vi "configMQTT.vi"(8 "error in (no error)":errorcluster, 10 "conf(empty for default)":string, 11 "Module ID":i32=-1) -> (0 "error out":errorcluster)   [LabVIEW 2017, in "ISA010_module.lvlib"]
uses:
  ISA010_module.lvlib
  libraries/MQTT.lvlibp
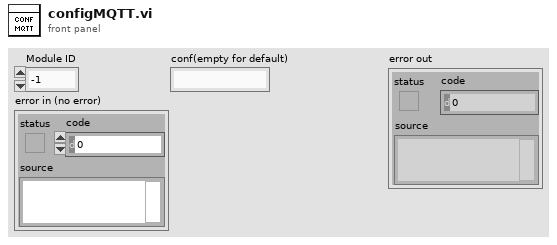
[diagram p1: front panel]
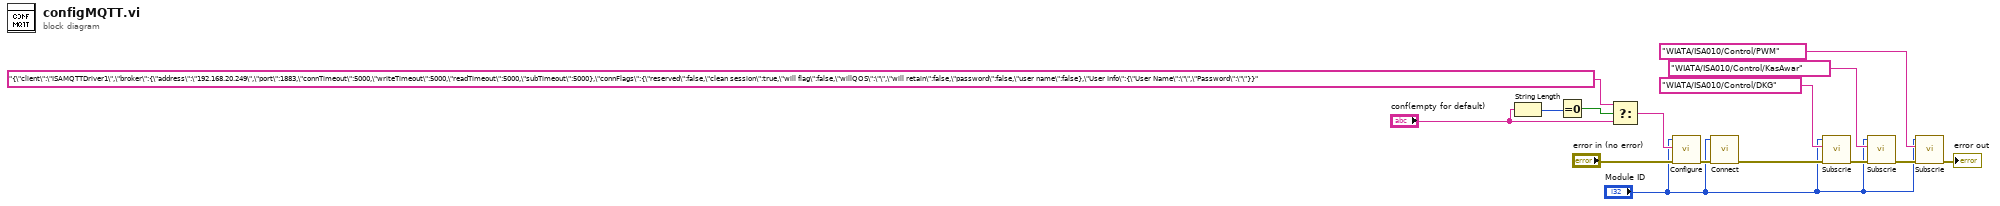
[diagram p0: block diagram]
diagram:
  n1 = String Length(string="conf(empty for default)") -> (length=w13:i32)
  n2 = Equal To 0?(x=w13) -> (x = 0?=w12:bool)
  n3 = Select(t="{\"client\":\"ISAMQTTDriver1\",\"broker\":{\"address\":\"192.168.20.249\",\"port\":1883,\"connTimeout\":5000,\"writeTimeout\":5000,\"readTimeout\":5000,\"subTimeout\":5000},\"connFlags\":{\"reserved\":false,\"clean session\":true,\"will flag\":false,\"willQOS\":\"\",\"will retain\":false,\"password\":false,\"user name\":false},\"User Info\":{\"User Name\":\"\",\"Password\":\"\"}}" ("JSON config"), s=w12, f="conf(empty for default)") -> (s? t:f=w9:string)
  n4 = call "Configure.vi"("error in (no error)"="error in (no error)", "JSON config"=w9, "Module ID"="Module ID") -> ("error out"=w15:errorcluster)  [unwired: 8 in]
  n5 = call "Connect.vi"("error in (no error)"=w15, "Module ID"="Module ID") -> ("error out"=w8:errorcluster)  [unwired: 9 in]
  n6 = call "Subscrie.vi"("error in (no error)"=w8, "String"="WIATA/ISA010/Control/DKG", "Module ID"="Module ID") -> ("error out"=w6:errorcluster)  [unwired: 8 in]
  n7 = call "Subscrie.vi"("error in (no error)"=w6, "String"="WIATA/ISA010/Control/KasAwar", "Module ID"="Module ID") -> ("error out"=w4:errorcluster)  [unwired: 8 in]
  n8 = call "Subscrie.vi"("error in (no error)"=w4, "String"="WIATA/ISA010/Control/PWM", "Module ID"="Module ID") -> ("error out"=→"error out":errorcluster)  [unwired: 8 in]
